vi "ExampleWriter.vi"() -> ()   [LabVIEW 2013]
uses:
  HelperVIs/EStopAction.ctl
  Writer/NetworkStreamWriter.lvclass
panel:
  out "Connected? 2":bool
  out "Connected?":bool
  out "Current iteration 2":i32
  in  "Cluster":T1
  out "Current iteration 1":i32
  in  "stop":bool
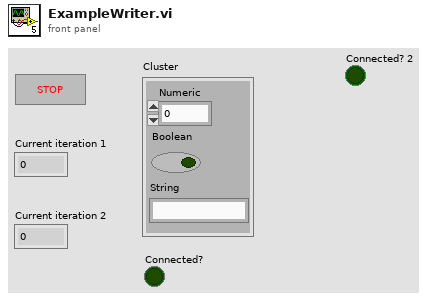
[diagram p1: front panel]
types:
  T1 = cluster{"Numeric":dbl, "Boolean":bool, "String":string}
  T2 = typedef "EStopAction.ctl" = enum16{"Get", "Set"}
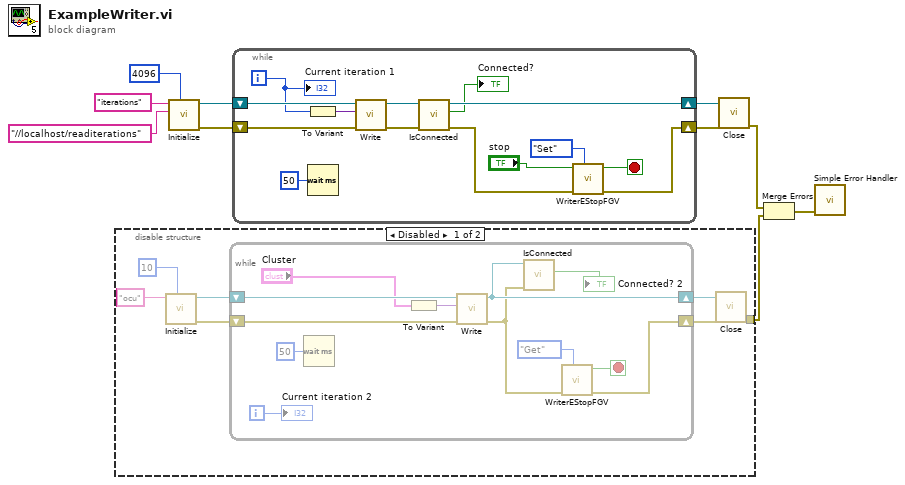
[diagram p0: block diagram]
diagram:
  n1 = disable-structure shown="Disabled" {
    disable-tunnel: [w12 _] -> w9
    frame Disabled {
      n2 = call "Initialize.vi"("writer buffer size"=10, "writer name"="ocu") -> ("error out"=w14:errorcluster, "NetworkStreamWriter out"=w13:refnum<class "NetworkStreamWriter.lvclass">)  [unwired: 8 in]
      n3 = while {
        shift-right: [w22] -> w17
        shift-left: w14 -> [w28]
        shift-right: [w21] -> w16
        shift-left: w13 -> [w29]
        i -> [w24]
        stop <- w18 stop-if-true
        n4 = Wait (ms)(milliseconds to wait=u32 50) -> ()  [unwired: 1 out]
        n5 = To Variant(anything="Cluster") -> (Variant=w27:variant)
        n6 = call "Write.vi"("error in (no error)"=w28, "element"=w27, "NetworkStreamWriter in"=w29) -> ("error out"=w20:errorcluster, "NetworkStreamWriter out"=w21:refnum<class "NetworkStreamWriter.lvclass">)  [unwired: 7 in]
        n7 = call "IsConnected.vi"("error in (no error)"=w20, "NetworkStreamWriter in"=w21) -> ("Connected?"=→"Connected? 2":bool)  [unwired: 7 in, 2 out]
        n8 = call "WriterEStopFGV.vi"("E-Stop Action"=EStopAction."Get", "Error In"=w20) -> ("Error Out"=w22:errorcluster, "E-Stop Out"=w18:bool)  [unwired: 8 in]
        "Current iteration 2" <- w24
      }
      n9 = call "Close.vi"("error in (no error)"=w17, "NetworkStreamWriter in"=w16) -> ("error out"=w12:errorcluster)  [unwired: 9 in]
    }
    frame Enabled {
    }
  }
  n10 = call "Initialize.vi"("writer buffer size"=4096, "reader url"="//localhost/readiterations" ("writer url"), "writer name"="iterations") -> ("error out"=w6:errorcluster, "NetworkStreamWriter out"=w7:refnum<class "NetworkStreamWriter.lvclass">)  [unwired: 7 in]
  n11 = while {
    shift-right: [w36] -> w3
    shift-left: w6 -> [w42]
    shift-right: [w33] -> w4
    shift-left: w7 -> [w43]
    i -> [w41]
    stop <- w37 stop-if-true
    n12 = To Variant(anything=w41) -> (Variant=w40:variant)
    n13 = Wait (ms)(milliseconds to wait=u32 50) -> ()  [unwired: 1 out]
    n14 = call "Write.vi"("error in (no error)"=w42, "element"=w40, "NetworkStreamWriter in"=w43) -> ("error out"=w34:errorcluster, "NetworkStreamWriter out"=w35:refnum<class "NetworkStreamWriter.lvclass">)  [unwired: 7 in]
    n15 = call "IsConnected.vi"("error in (no error)"=w34, "NetworkStreamWriter in"=w35) -> ("error out"=w32:errorcluster, "Connected?"=→"Connected?":bool, "NetworkStreamWriter out"=w33:refnum<class "NetworkStreamWriter.lvclass">)  [unwired: 7 in]
    n16 = call "WriterEStopFGV.vi"("E-Stop Action"=EStopAction."Set", "Error In"=w32, "E-Stop In"="stop") -> ("Error Out"=w36:errorcluster, "E-Stop Out"=w37:bool)  [unwired: 7 in]
    "Current iteration 1" <- w41
  }
  n17 = call "Close.vi"("error in (no error)"=w3, "NetworkStreamWriter in"=w4) -> ("error out"=w10:errorcluster)  [unwired: 9 in]
  n18 = Merge Errors(w10, w9) -> (w8:errorcluster)
  n19 = call <vilib>:"Simple Error Handler.vi"("error in (no error)"=w8) -> ()  [unwired: 4 in, 5 out]
